vi "disable.vi"(8 "error in (no error)":errorcluster, 10 "model in":refnum<class "IModel.lvclass">, 11 "NotImagingState in":refnum<class "NotImagingState.lvclass">) -> (0 "error out":errorcluster, 2 "model out":refnum<class "IModel.lvclass">, 3 "NotImagingState out":refnum<class "NotImagingState.lvclass">)   [LabVIEW 2016, in "States.lvlib" / "NotImagingState.lvclass"]
uses:
  NotImagingState.lvclass
  IModel/IModel.lvclass
  Typedefs/CommandValue.ctl
  Typedefs/SEDSpectrometerTypedefs.lvlib
  ts_sallv_FiberSpectrograph/DataTypes/logevent_detailedState.ctl
  ts_sallv_FiberSpectrograph/SALLV_FiberSpectrograph.lvlib
  ts_sallv_FiberSpectrograph/DataTypes/logevent_summaryState.ctl
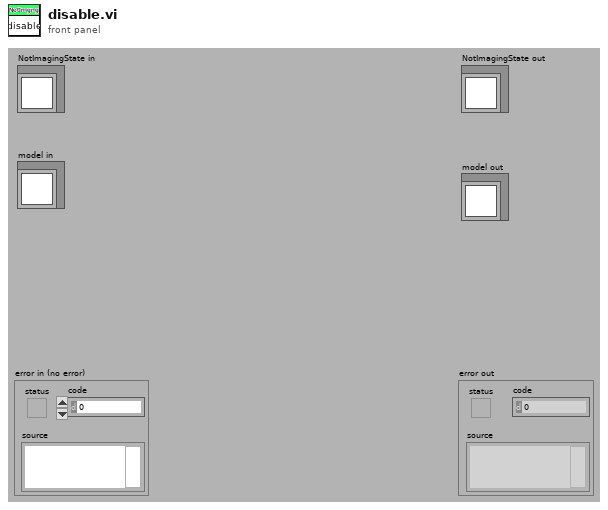
[diagram p1: front panel]
types:
  T1 = typedef "SALLV_FiberSpectrograph.lvlib/logevent_summaryState.ctl" = cluster{"summaryState":i32, "priority":i32}
  T2 = typedef "SALLV_FiberSpectrograph.lvlib/logevent_detailedState.ctl" = cluster{"detailedState":i32, "priority":i32}
  T3 = typedef "SEDSpectrometerTypedefs.lvlib/CommandValue.ctl" = enum16{"clearError", "disable", "enable", "exit", "GoToStandby", "OnHeartbeat", "OnIncomingMessagingError", "OnInterrupt", "start", "captureSpectImage", "setSpectTempSetpoint", "stopImageCapture"}
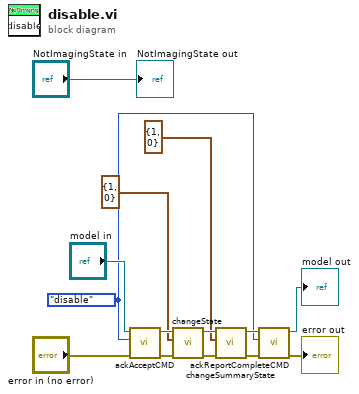
[diagram p0: block diagram]
diagram:
  w3 = CommandValue."disable" ("CommandValue")
  n1 = call-dynamic "ackAcceptCMD.vi"("error in (no error)"="error in (no error)", "CommandValue"=w3, "IModel in"="model in") -> ("error out"=w11:errorcluster, "IModel out"=w8:refnum<class "IModel.lvclass">)  [unwired: 7 in]
  n2 = call-dynamic "changeState.vi"("error in (no error)"=w11, "DetailedState"=T2 {"detailedState"=1, "priority"=0}, "IModel in"=w8) -> ("error out"=w10:errorcluster, "IModel out"=w9:refnum<class "IModel.lvclass">)  [unwired: 7 in]
  n3 = call-dynamic "changeSummaryState.vi"("error in (no error)"=w10, "logevent_SummaryState"=T1 {"summaryState"=1, "priority"=0}, "IModel in"=w9) -> ("error out"=w5:errorcluster, "IModel out"=w4:refnum<class "IModel.lvclass">)  [unwired: 7 in]
  n4 = call-dynamic "ackReportCompleteCMD.vi"("error in (no error)"=w5, "CommandValue"=w3, "IModel in"=w4) -> ("error out"=→"error out":errorcluster, "IModel out"=→"model out":refnum<class "IModel.lvclass">)  [unwired: 7 in]
  "NotImagingState out" <- "NotImagingState in"
